vi "in_2d interp prepare arrays.vi"(0 "size of Z":i32[](array[numeric]), 5 "X":dbl[][](array[numeric]), 7 "Y":dbl[][](array[numeric]), 9 "xi size":i32[](array[numeric]), 11 "yi size":i32[](array[numeric]), 12 "ntimes":i32=1) -> (3 "new size of Z":i32[](array[numeric]), 4 "X-out":dbl[](array[numeric]), 6 "Y-out":dbl[](array[numeric]), 14 "ntimes remaining":i32=1, 15 "error":i32)   [LabVIEW 2010, in "NI_Gmath.lvlib"]
uses:
  NI_Gmath.lvlib
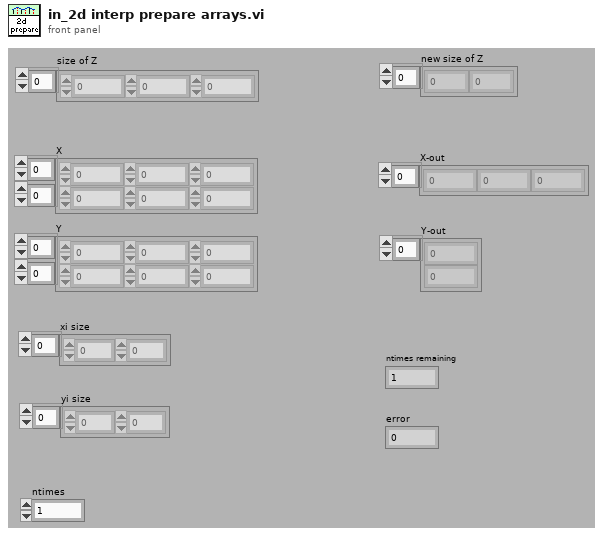
[diagram p1: front panel]
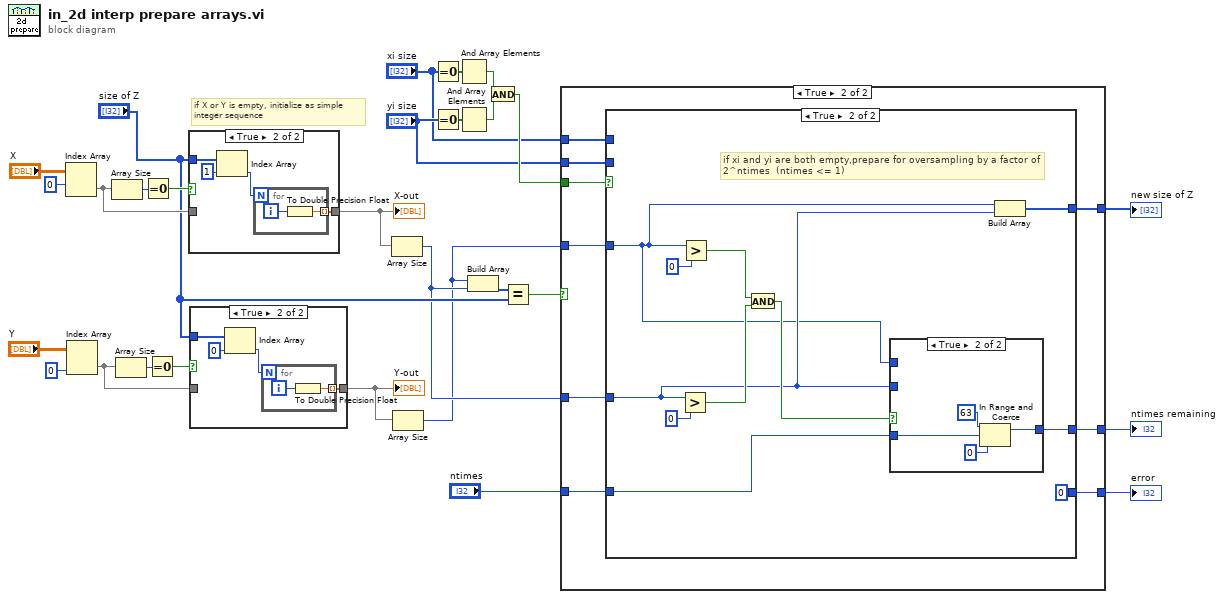
[diagram p0: block diagram]
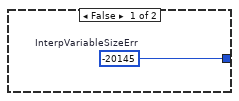
[diagram p2: hidden frame]
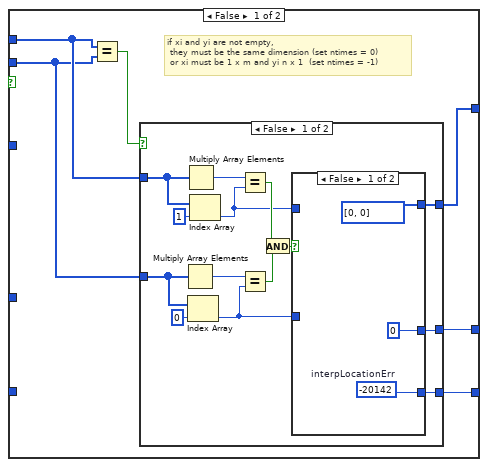
[diagram p3: hidden frame]
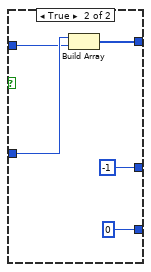
[diagram p4: hidden frame]
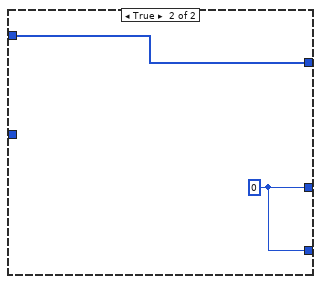
[diagram p5: hidden frame]
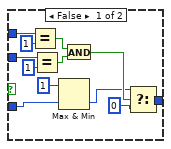
[diagram p6: hidden frame]
diagram:
  # "if X or Y is empty, initialize as simple\ninteger sequence"
  n1 = Index Array(array="X", index (row)=0) -> (element=w25:dbl[])  [unwired: 1 in]
  n2 = Index Array(array="Y", index (col)=0 ("index (row)")) -> (element=w20:dbl[])  [unwired: 1 in]
  n3 = Array Size(array=w25) -> (size(s)=w24:i32)
  n4 = Array Size(array=w20) -> (size(s)=w22:i32)
  n5 = Equal To 0?(x=w24) -> (x = 0?=w23:bool)
  n6 = Equal To 0?(x=w22) -> (x = 0?=w21:bool)
  n7 = case shown="True" w23 {
    tunnel: w25 -> [w29 _]
    tunnel: [w29 w32] -> w11
    tunnel: "size of Z" -> [_ w31]
    frame False {
    }
    frame True {
      n8 = Index Array(array=w31, index=1 ("index (row)")) -> (element=w30:i32)
      n9 = for {
        N: w30 -> [_]
        tunnel: [w34] -> w32 mode=indexing
        i -> [w35]
        n10 = To Double Precision Float(number=w35) -> (double precision float=w34:dbl)
      }
    }
  }
  "X-out" <- w11
  n11 = case shown="True" w21 {
    tunnel: w20 -> [w36 _]
    tunnel: [w36 w40] -> w10
    tunnel: "size of Z" -> [_ w39]
    frame False {
    }
    frame True {
      n12 = Index Array(array=w39, index=0 ("index (row)")) -> (element=w37:i32)
      n13 = for {
        N: w37 -> [_]
        tunnel: [w41] -> w40 mode=indexing
        i -> [w42]
        n14 = To Double Precision Float(number=w42) -> (double precision float=w41:dbl)
      }
    }
  }
  "Y-out" <- w10
  n15 = Array Size(array=w11) -> (size(s)=w2:i32)
  n16 = Array Size(array=w10) -> (size(s)=w1:i32)
  n17 = Equal To 0?(x="xi size") -> (x = 0?=w19:bool[])
  n18 = Equal To 0?(x="yi size") -> (x = 0?=w18:bool[])
  n19 = And Array Elements(Boolean array=w19) -> (logical AND=w16:bool)
  n20 = And Array Elements(Boolean array=w18) -> (logical AND=w15:bool)
  n21 = Build Array(w1, w2) -> (w4:i32[])
  n22 = And(x=w16, y=w15) -> (x .and. y?=w14:bool)
  n23 = Equal?(x=w4, y="size of Z") -> (x = y?=w3:bool)
  n24 = case shown="True" w3 {
    tunnel: w14 -> [_ w52]
    tunnel: "ntimes" -> [_ w51]
    tunnel: [_ w50] -> w12
    tunnel: w1 -> [_ w49]
    tunnel: w2 -> [_ w48]
    tunnel: [w43 w47] -> w9
    tunnel: "yi size" -> [_ w46]
    tunnel: "xi size" -> [_ w45]
    tunnel: [_ w44] -> w6
    frame False {
      w43 = -20145  # InterpVariableSizeErr
    }
    frame True {
      n25 = case shown="True" w52 {
        tunnel: w51 -> [_ w90]
        tunnel: [w57 w93] -> w50
        tunnel: w49 -> [_ w84]
        tunnel: w48 -> [_ w85]
        tunnel: [w56 0 ("error")] -> w47
        tunnel: w46 -> [w54 _]
        tunnel: w45 -> [w55 _]
        tunnel: [w53 w83] -> w44
        frame False {
          # "if xi and yi are not empty,\n they must be the same dimension (set ntimes = 0)\n or xi must be 1 x m and yi n x 1  (set ntimes = -1)"
          n26 = Equal?(x=w55, y=w54) -> (x = y?=w58:bool)
          n27 = case shown="False" w58 {
            tunnel: [w64 w82] -> w57
            tunnel: [w65 w82] -> w56
            tunnel: w55 -> [w66 w81]
            tunnel: w54 -> [w61 _]
            tunnel: [w63 w81] -> w53
            frame False {
              n28 = Multiply Array Elements(1:w61) -> (0:w70:i32)
              n29 = Multiply Array Elements(1:w66) -> (0:w71:i32)
              n30 = Index Array(array=w61, index=0) -> (element=w60:i32)
              n31 = Index Array(array=w66, index=1) -> (element=w59:i32)
              n32 = Equal?(x=w71, y=w59) -> (x = y?=w69:bool)
              n33 = Equal?(x=w70, y=w60) -> (x = y?=w68:bool)
              n34 = And(x=w69, y=w68) -> (x .and. y?=w67:bool)
              n35 = case shown="False" w67 {
                tunnel: [w73 0 ("t")] -> w65
                tunnel: [0 ("t") -1] -> w64
                tunnel: [i32[] [0, 0] ("new size of Z") w76] -> w63
                tunnel: w60 -> [_ w78]
                tunnel: w59 -> [_ w77]
                frame False {
                  w73 = -20142  # interpLocationErr
                }
                frame True {
                  n36 = Build Array(w78, w77) -> (w76:i32[])
                }
              }
            }
            frame True {
              w82 = 0 ("upper limit")
            }
          }
        }
        frame True {
          # "if xi and yi are both empty,prepare for oversampling by a factor of\n2^ntimes  (ntimes <= 1)"
          n37 = Greater?(x=w85, y=0 ("upper limit")) -> (0:w87:bool)
          n38 = Greater?(x=w84, y=0 ("upper limit")) -> (0:w88:bool)
          n39 = And(x=w88, y=w87) -> (x .and. y?=w89:bool)
          n40 = case shown="True" w89 {
            tunnel: [w98 w107] -> w93
            tunnel: w90 -> [w94 w106]
            tunnel: w84 -> [w104 _]
            tunnel: w85 -> [w101 _]
            frame False {
              n41 = Equal?(x=w104, y=1) -> (x = y?=w100:bool)
              n42 = Equal?(x=w101, y=1) -> (x = y?=w99:bool)
              n43 = Max & Min(x=1 ("t"), y=w94) -> (min(x,y)=w95:i32)  [unwired: 1 out]
              n44 = And(x=w100, y=w99) -> (x .and. y?=w97:bool)
              n45 = Select(t=w95, s=w97, f=0 ("upper limit")) -> (s? t:f=w98:i32)
            }
            frame True {
              n46 = In Range and Coerce(upper limit=63, x=w106, lower limit=0 ("upper limit")) -> (coerced(x)=w107:i32)  [unwired: 1 out]
            }
          }
          n47 = Build Array(w84, w85) -> (w83:i32[])
        }
      }
    }
  }
  "ntimes remaining" <- w12
  "new size of Z" <- w6
  "error" <- w9
